vi "database_connection_write_dev_MQTT_database_array_V1.vi"(8 "error in (no error)":errorcluster, 9 "data 2":dbl[](array[numeric]), 10 "Machine Data":T5={"Zload"="", "Yload"="", "Xload"="", "path_position"="", "Fovr"="", "SspeedOvr"="", "Program Name"="", "Program status"="", "Block of code being executed"="", "Line of code"="", "Machine availability"="", "Emergency status"="", "Controller mode"="", "Tool_id"="UNAVAILABLE"}, 11 "current time 2":timestamp) -> (3 "error out":errorcluster)   [LabVIEW 2017]
uses:
  mqtt Folder/src/class/mqtt/mqttTypedef/mqttConnectionStatus.ctl
  mqtt Folder/src/class/mqtt/mqttTypedef/mqttConnectionMeta.ctl
  mqtt Folder/src/class/mqtt/mqttTypedef/mqttQOSlevel.ctl
  data_base_structure_V2.ctl
  mqtt Folder/src/class/mqtt/mqttConfigFunction.ctl
  mqtt Folder/src/class/mqtt/mqttTypedef/mqttBroker.ctl
  mqtt Folder/src/class/mqtt/mqttTypedef/mqttConnectionFlags.ctl
  mqtt Folder/src/class/mqtt/mqttTypedef/mqttWillInformation.ctl
  mqtt Folder/src/class/mqtt/mqttTXqueue/mqttTXdataQueueFunction.ctl
  mqtt Folder/src/class/mqtt/mqttTXqueue/mqttRXsubscriptionEventFunction.ctl
  data_base_structure.ctl
  <vilib>/addons/database/Connection.llb/DB Tools Open Connec (Path).vi
  mqtt Folder/src/class/mqtt/mqtt.lvclass
  <vilib>/addons/database/NI_Database_API.lvlib
panel:
  out "cluster":T1
  out "Xload":string
  out "Machine availability":string
  out "resulting string":string
  out "output array 2":dbl[](array[numeric])
  out "size(s) 2":i32
  out "error out 3":errorcluster
  out "publishSuccess 2":bool=TRUE
  out "publishMessageID 2":u16 format="%02x"
  out "valueSent 2":string="14:19:17.238_"
  in  "connMeta 2":T2
  in  "topic 2":string="a/b"
  out "connStatus 2":T4
  out "sessionPresent 2":bool
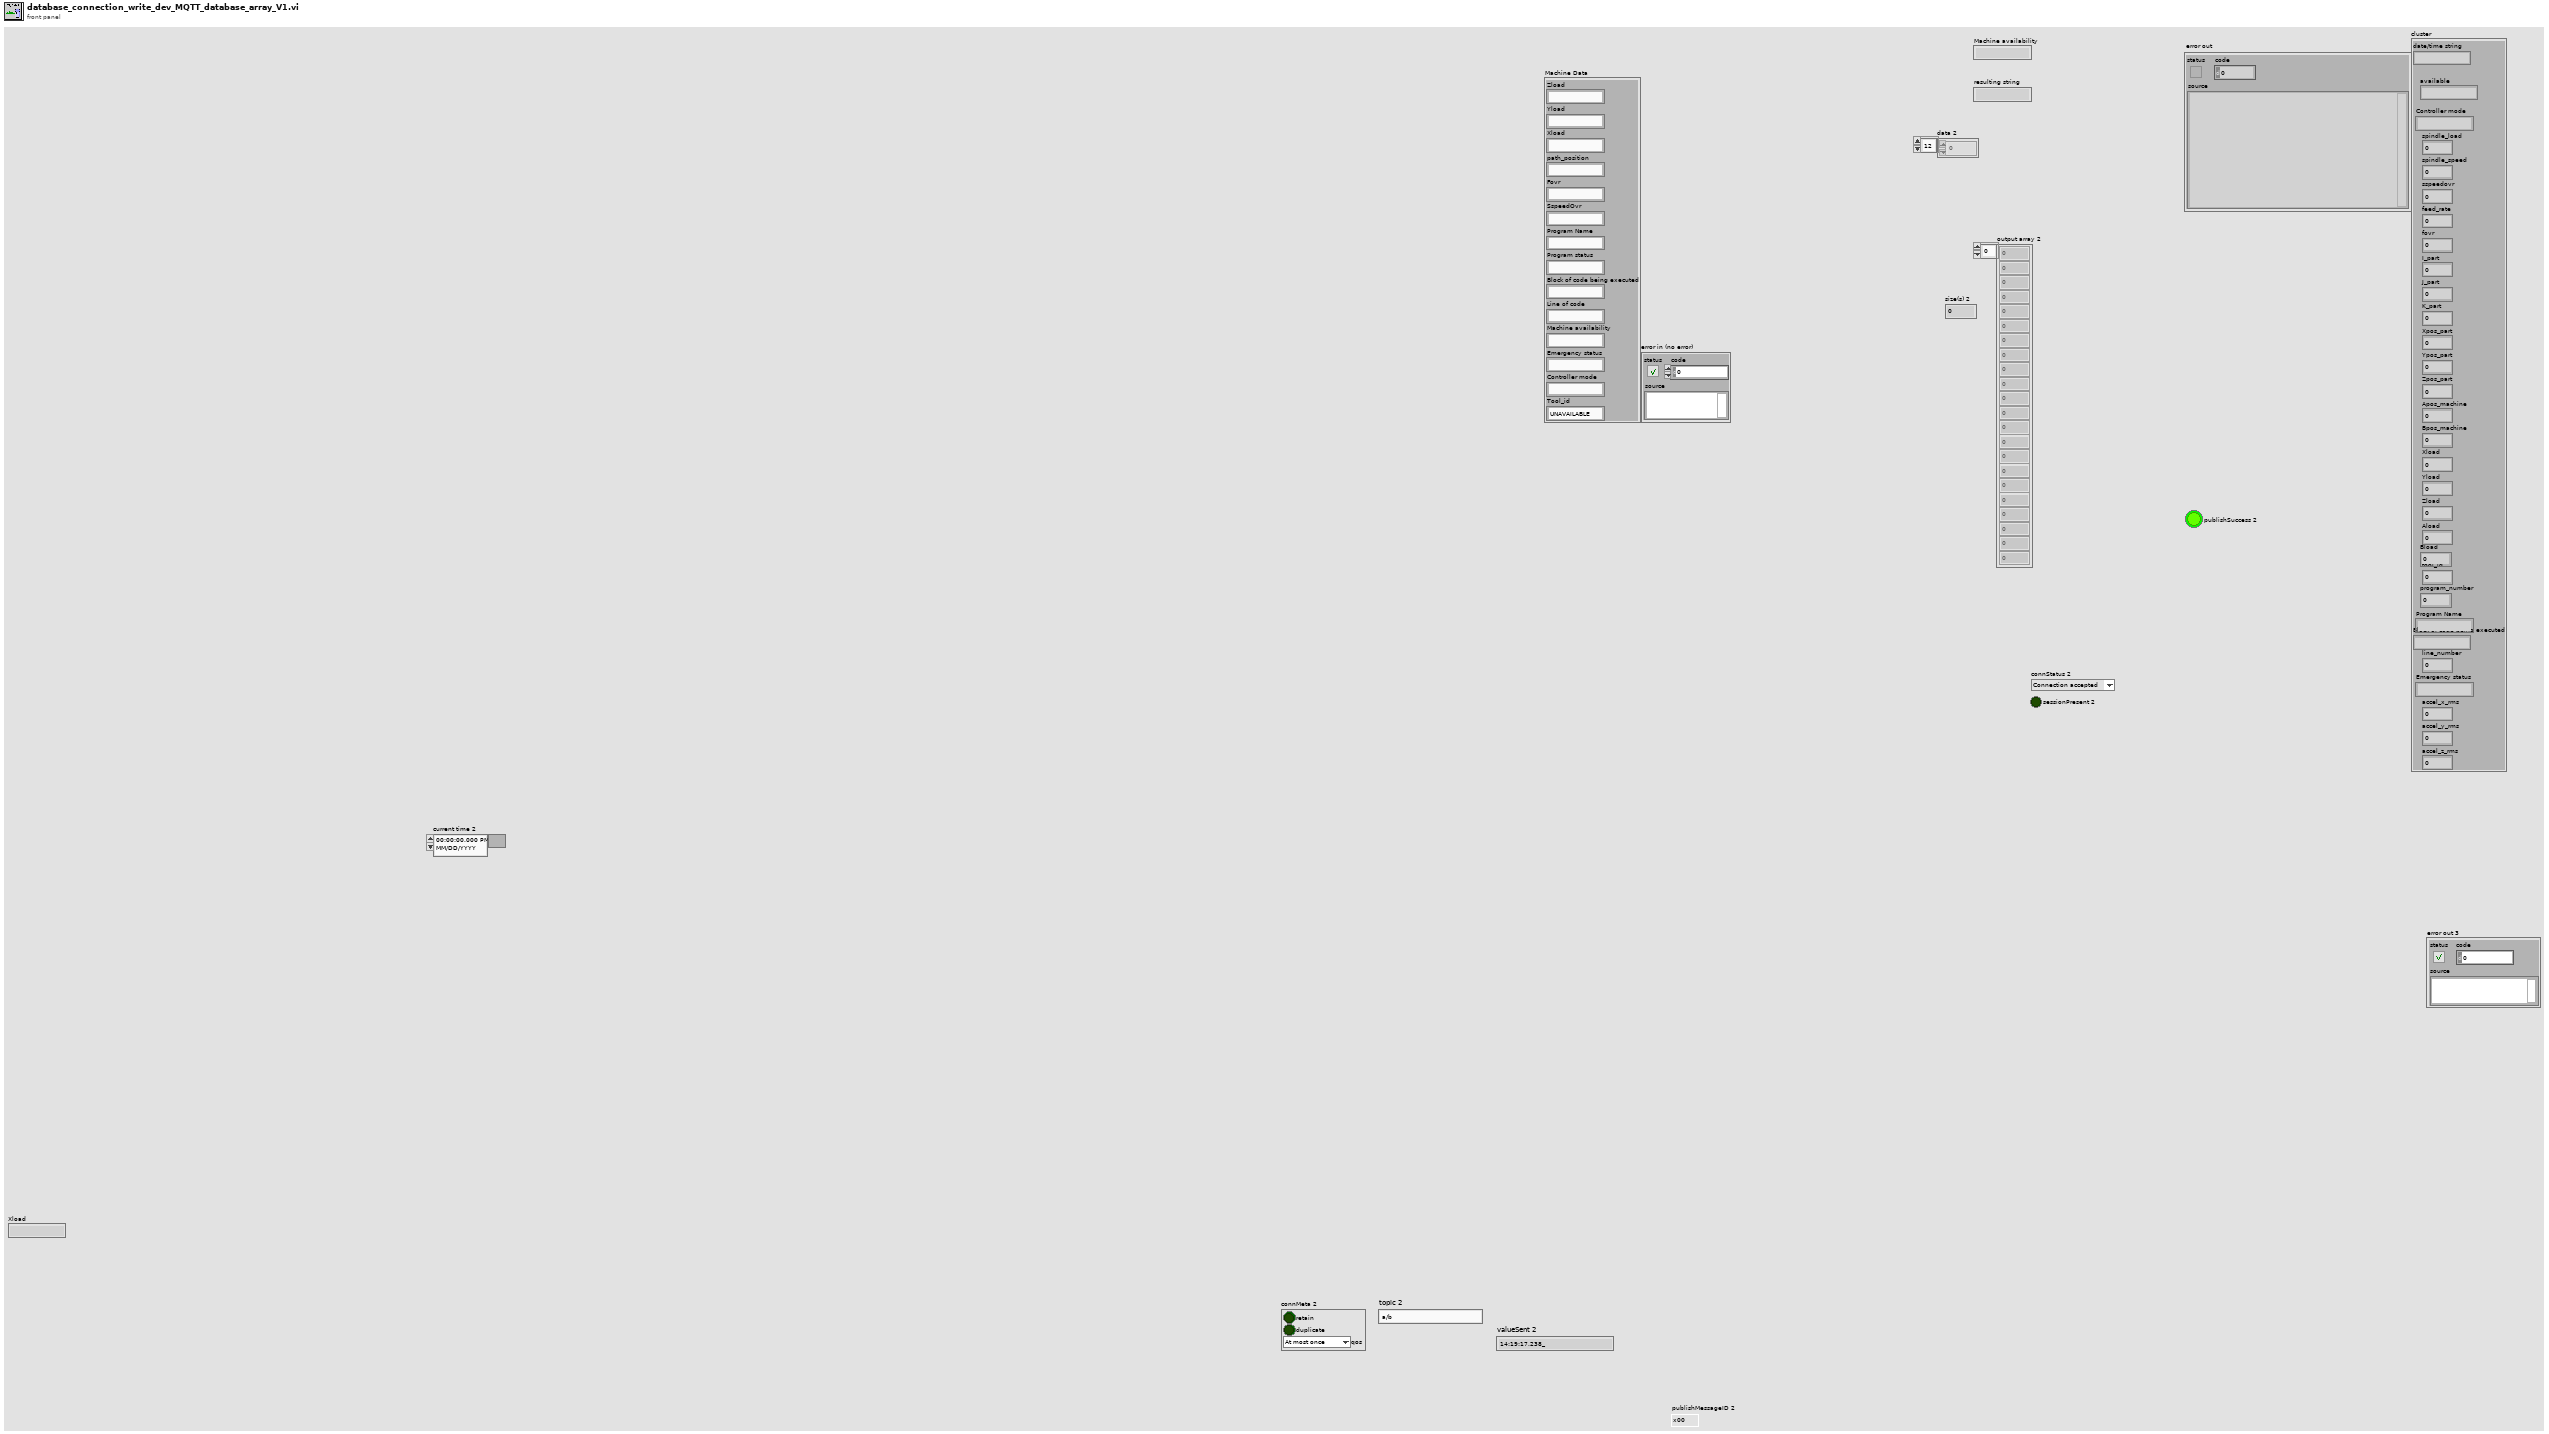
[diagram p1: front panel]
types:
  T1 = typedef "data_base_structure_V2.ctl" = cluster{"date/time string":string, "available":string, "Controller mode":string, "spindle_load":dbl, "spindle_speed":dbl, "sspeedovr":dbl, "feed_rate":dbl, "fovr":dbl, "I_part":dbl, "J_part":dbl, "K_part":dbl, "Xpos_part":dbl, "Ypos_part":dbl, "Zpos_part":dbl, "Apos_machine":dbl, "Bpos_machine":dbl, "Xload":dbl, "Yload":dbl, "Zload":dbl, "Aload":dbl, "Bload":dbl, "tool_id":dbl, "program_number":dbl, "Program Name":string, "Block of code being executed":string, "line_number":dbl, "Emergency status":string, "accel_x_rms":dbl, "accel_y_rms":dbl, "accel_z_rms":dbl}
  T2 = typedef "mqttConnectionMeta.ctl" = cluster{"retain":bool, "duplicate":bool, "qos":T3}
  T3 = typedef "mqttQOSlevel.ctl" = enum8{"At most once", "At least once", "Exactly once", "Reserved"}
  T4 = typedef "mqttConnectionStatus.ctl" = enum16{"Connection accepted", "Connection refused: unacceptable protocol version", "Connection refused: identifier rejected", "Connection refused: Server unavailable", "Connection refused: bad user name or password", "Connection refused: not authorized"}
  T5 = cluster{"Zload":string, "Yload":string, "Xload":string, "path_position":string, "Fovr":string, "SspeedOvr":string, "Program Name":string, "Program status":string, "Block of code being executed":string, "Line of code":string, "Machine availability":string, "Emergency status":string, "Controller mode":string, "Tool_id":string}
  T6 = typedef "data_base_structure.ctl" = cluster{"available ":dbl, "controller_mode":string, "spindle_load":dbl, "spindle_speed ":dbl, "sspeedovr":dbl, "J_part":dbl, "K_part":dbl, "Xpos_part":dbl, "Ypos_part":dbl, "Zpos_part":dbl, "Apos_machine":dbl, "Bpos_machine":dbl, "Xload":dbl, "Yload":dbl, "Zload":dbl, "Aload":dbl, "Bload":dbl, "tool_id":dbl, "program_name":string, "block_code":string, "line_number":dbl, "estop":string, "accel_x_rms":dbl, "accel_y_rms":dbl, "accel_z_rms":dbl, "program_number":dbl, "timestamp":string, "feed_rate ":dbl, "fovr":dbl, "I_part ":dbl}
  T7 = typedef "mqttRXsubscriptionEventFunction.ctl" = enum16{"init", "deinit", "getEventRef", "event"}
  T8 = typedef "mqttTXdataQueueFunction.ctl" = enum16{"init", "deinit", "getQueue", "enqueue"}
  T9 = typedef "mqttWillInformation.ctl" = cluster{"User Name":string, "Password":string}
  T10 = typedef "mqttConnectionFlags.ctl" = cluster{"reserved":bool, "clean session":bool, "will flag":bool, "willQOS":enum8{"At most once", "At least once", "Exactly once", "Reserved"}, "will retain":bool, "password":bool, "user name":bool}
  T11 = typedef "mqttBroker.ctl" = cluster{"address":string, "port":u16, "connTimeout":i32, "writeTimeout":i32, "readTimeout":i32, "subTimeout":i32}
  T12 = typedef "mqtt.lvclass/mqttConfigFunction.ctl" = enum16{"init", "deinit", "set", "get"}
  T13 = enum8{"Enabled", "Disabled", "Disabled and Grayed Out"}
  T14 = cluster{"data 2[0]":dbl, "data 2[1]":dbl, "data 2[2]":dbl, "data 2[3]":dbl, "data 2[4]":dbl, "data 2[5]":dbl, "data 2[6]":dbl, "data 2[7]":dbl, "data 2[8]":dbl, "data 2[9]":dbl, "data 2[10]":dbl, "data 2[11]":dbl, "data 2[12]":dbl, "data 2[13]":dbl, "data 2[14]":dbl, "data 2[15]":dbl, "data 2[16]":dbl, "data 2[17]":dbl, "data 2[18]":dbl, "data 2[19]":dbl, "data 2[20]":dbl, "data 2[21]":dbl}
  T15 = typedef "NI_Database_API.lvlib/Conn ObjectReference.ctl" = refnum<k1>
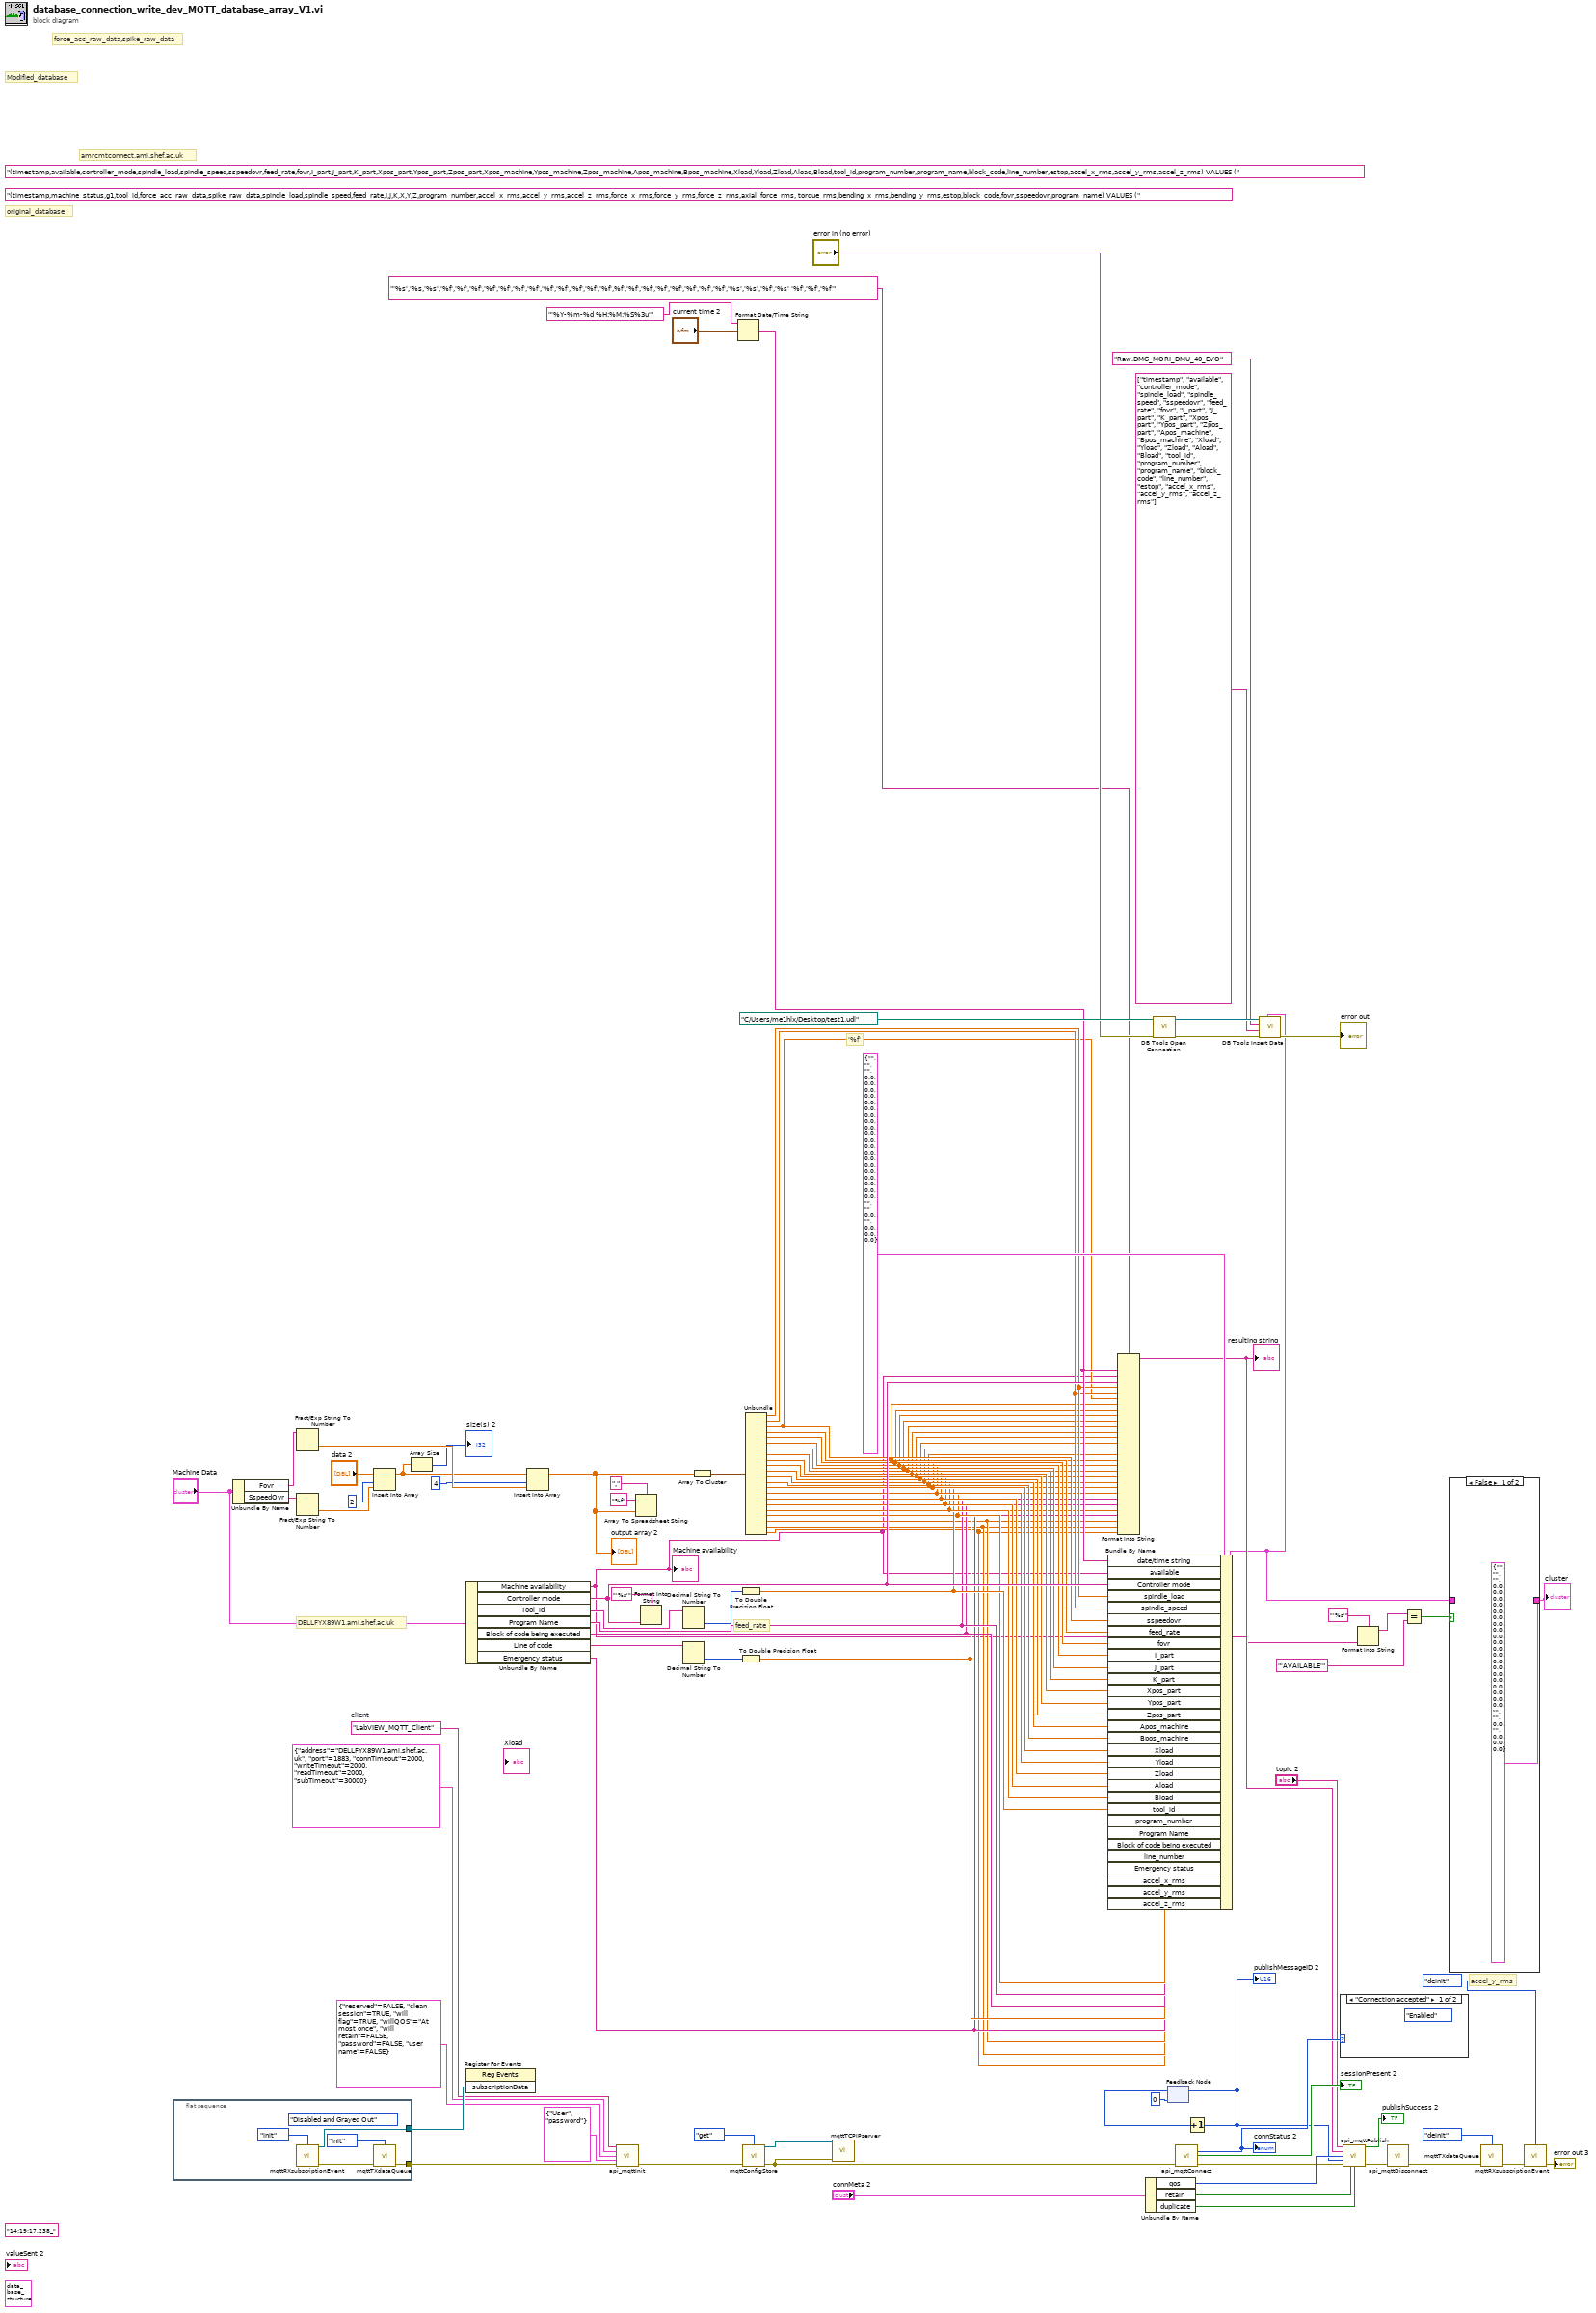
[diagram p0: block diagram]
diagram:
  (unwired) "14:19:17.238_" ("valueSent 2")
  (unwired) T6 {"available "=0.0, "controller_mode"="", "spindle_load"=0.0, "spindle_speed "=0.0, "sspeedovr"=0.0, "J_part"=0.0, "K_part"=0.0, "Xpos_part"=0.0, "Ypos_part"=0.0, "Zpos_part"=0.0, "Apos_machine"=0.0, "Bpos_machine"=0.0, "Xload"=0.0, "Yload"=0.0, "Zload"=0.0, "Aload"=0.0, "Bload"=0.0, "tool_id"=0.0, "program_name"="", "block_code"="", "line_number"=0.0, "estop"="", "accel_x_rms"=0.0, "accel_y_rms"=0.0, "accel_z_rms"=0.0, "program_number"=0.0, "timestamp"="", "feed_rate "=0.0, "fovr"=0.0, "I_part "=0.0} ("Cluster")
  (unwired) "(timestamp,available,controller_mode,spindle_load,spindle_speed,sspeedovr,feed_rate,fovr,I_part,J_part,K_part,Xpos_part,Ypos_part,Zpos_part,Xpos_machine,Ypos_machine,Zpos_machine,Apos_machine,Bpos_machine,Xload,Yload,Zload,Aload,Bload,tool_id,program_number,program_name,block_code,line_number,estop,accel_x_rms,accel_y_rms,accel_z_rms) VALUES (" ("string")
  w88 = "LabVIEW_MQTT_Client"  # client
  (unwired) "(timestamp,machine_status,g1,tool_id,force_acc_raw_data,spike_raw_data,spindle_load,spindle_speed,feed_rate,I,J,K,X,Y,Z,program_number,accel_x_rms,accel_y_rms,accel_z_rms,force_x_rms,force_y_rms,force_z_rms,axial_force_rms, torque_rms,bending_x_rms,bending_y_rms,estop,block_code,fovr,sspeedovr,program_name) VALUES (" ("string")
  # "'%f'"
  # "accel_y_rms"
  # "feed_rate"
  # "original_database"
  # "force_acc_raw_data,spike_raw_data"
  # "Modified_database"
  # "amrcmtconnect.ami.shef.ac.uk"
  # "DELLFYX89W1.ami.shef.ac.uk"
  n1 = flat-sequence {
    tunnel: [w99] -> w93
    tunnel: [w96] -> w89
    frame #0 {
      (unwired) T13."Disabled and Grayed Out" ("Disabled")
      n2 = call "mqttRXsubscriptionEvent.vi"("function"=mqttRXsubscriptionEventFunction."init") -> ("subscriptionData"=w96:refnum<user-event>, "error out"=w98:errorcluster)  [unwired: 13 in]
      n3 = call "mqttTXdataQueue.vi"("function"=mqttTXdataQueueFunction."init", "error in (no error)"=w98) -> ("error out"=w99:errorcluster)  [unwired: 12 in, 1 out]
    }
  }
  n4 = Unbundle By Name("Machine Data") -> ("Fovr"=w59:string, "SspeedOvr"=w64:string)
  n5 = Fract/Exp String To Number(string=w59) -> (number=w61:dbl)  [unwired: 3 in, 1 out]
  n6 = Fract/Exp String To Number(string=w64) -> (number=w63:dbl)  [unwired: 3 in, 1 out]
  n7 = Insert Into Array(array="data 2", index=2, new element=w63) -> (w52:dbl[])
  n8 = Array Size(array=w52) -> (size(s)=→"size(s) 2":i32)
  n9 = Unbundle By Name("Machine Data") -> ("Machine availability"=w5:string, "Controller mode"=w37:string, "Tool_id"=w49:string, "Program Name"=w16:string, "Block of code being executed"=w15:string, "Line of code"=w48:string, "Emergency status"=w13:string)
  "Machine availability" <- w5
  n10 = register-events(w89) -> ()  [unwired: 2 in, 2 out]
  n11 = Insert Into Array(array=w52, index=4, new element=w61) -> (w42:dbl[])
  "output array 2" <- w42
  n12 = call "api_mqttInit.vi"("client"=w88, "broker"=T11 {"address"="DELLFYX89W1.ami.shef.ac.uk", "port"=1883, "connTimeout"=2000, "writeTimeout"=2000, "readTimeout"=2000, "subTimeout"=30000}, "connFlags"=T10 {"reserved"=FALSE, "clean session"=TRUE, "will flag"=TRUE, "willQOS"=enum."At most once", "will retain"=FALSE, "password"=FALSE, "user name"=FALSE}, "User Info"=T9 {"User Name"="User", "Password"="password"}, "error in (no error)"=w93) -> ("error out"=w91:errorcluster)  [unwired: 10 in]
  n13 = Array To Spreadsheet String(delimiter (Tab)=",", array=w42, 3:"%f" ("format string")) -> ()  [unwired: 1 out]
  n14 = Format Into String(format string="'%s'", w37) -> ()  [unwired: 2 in, 2 out]
  n15 = Decimal String To Number(string=w49) -> (number=w50:i32)  [unwired: 2 in, 1 out]
  n16 = Decimal String To Number(string=w48) -> (number=w47:i32)  [unwired: 2 in, 1 out]
  n17 = Array To Cluster(array=w42) -> (cluster=w41:T14)
  n18 = Format Date/Time String(time format string (%c)="'%Y-%m-%d %H:%M:%S%3u'", seconds (now)="current time 2") -> (date/time string=w38:string)  [unwired: 1 in]
  n19 = To Double Precision Float(number=w50) -> (double precision float=w18:dbl)
  n20 = To Double Precision Float(number=w47) -> (double precision float=w14:dbl)
  n21 = call "mqttConfigStore.vi"("function"=mqttConfigFunction."get", "error in (no error)"=w91) -> ("mqtt.lvclass out"=w90:refnum<class "mqtt.lvclass">, "error out"=w82:errorcluster)  [unwired: 12 in]
  n22 = Unbundle(w41) -> ("data 2[0]"=w36:dbl, "data 2[1]"=w35:dbl, "data 2[2]"=w34:dbl, "data 2[3]"=w33:dbl, "data 2[4]"=w32:dbl, "data 2[5]"=w31:dbl, "data 2[6]"=w30:dbl, "data 2[7]"=w29:dbl, "data 2[8]"=w28:dbl, "data 2[9]"=w27:dbl, "data 2[10]"=w26:dbl, "data 2[11]"=w25:dbl, "data 2[12]"=w24:dbl, "data 2[13]"=w23:dbl, "data 2[14]"=w22:dbl, "data 2[15]"=w21:dbl, "data 2[16]"=w20:dbl, "data 2[17]"=w19:dbl, "data 2[18]"=w17:dbl, "data 2[19]"=w11:dbl, "data 2[20]"=w10:dbl, "data 2[21]"=w9:dbl)
  n23 = call "mqttTCPIPserver.vi"("mqtt.lvclass"=w90, "error in (no error)"=w82) -> ()  [unwired: 12 in, 2 out]
  n24 = Bundle By Name(cluster=T1 {"date/time string"="", "available"="", "Controller mode"="", "spindle_load"=0.0, "spindle_speed"=0.0, "sspeedovr"=0.0, "feed_rate"=0.0, "fovr"=0.0, "I_part"=0.0, "J_part"=0.0, "K_part"=0.0, "Xpos_part"=0.0, "Ypos_part"=0.0, "Zpos_part"=0.0, "Apos_machine"=0.0, "Bpos_machine"=0.0, "Xload"=0.0, "Yload"=0.0, "Zload"=0.0, "Aload"=0.0, "Bload"=0.0, "tool_id"=0.0, "program_number"=0.0, "Program Name"="", "Block of code being executed"="", "line_number"=0.0, "Emergency status"="", "accel_x_rms"=0.0, "accel_y_rms"=0.0, "accel_z_rms"=0.0}, "date/time string"=w38, "available"=w5, "Controller mode"=w37, "spindle_load"=w36, "spindle_speed"=w35, "sspeedovr"=w34, "feed_rate"=w33, "fovr"=w32, "I_part"=w31, "J_part"=w30, "K_part"=w29, "Xpos_part"=w28, "Ypos_part"=w27, "Zpos_part"=w26, "Apos_machine"=w25, "Bpos_machine"=w24, "Xload"=w23, "Yload"=w22, "Zload"=w21, "Aload"=w20, "Bload"=w19, "tool_id"=w18, "program_number"=w17, "Program Name"=w16, "Block of code being executed"=w15, "line_number"=w14, "Emergency status"=w13, "accel_x_rms"=w11, "accel_y_rms"=w10, "accel_z_rms"=w9) -> (w2:T1)
  n25 = Format Into String(format string="'%s','%s,'%s','%f','%f','%f','%f','%f','%f','%f','%f','%f','%f','%f','%f',%f','%f','%f','%f','%f','%f','%f','%f','%s','%s','%f','%s' '%f','%f','%f'", w38, w5, w37, w36, w35, w34, w33, w32, w31, w30, w29, w28, w27, w26, w25, w24, w23, w22, w21, w20, w19, w18, w17, w16, w15, w14, w13, w11, w10, w9) -> (resulting string=w8:string)  [unwired: 2 in, 1 out]
  "resulting string" <- w8
  n26 = Unbundle By Name("connMeta 2") -> ("qos"=w79:T3, "retain"=w78:bool, "duplicate"=w77:bool)
  n27 = call-poly <vilib>:"DB Tools Open Connection.vi"("error in (no error)"="error in (no error)", "connection information"=path "C:/Users/me1hlx/Desktop/test1.udl") -> ("error out"=w51:errorcluster, "connection reference"=w56:T15)  [unwired: 6 in]
  n28 = feedback #1(u16 0) -> (w74:u16)
  n29 = call "api_mqttConnect.vi"("error in (no error)"=w82) -> ("connStatus"=w84:T4, "sessionPresent"=→"sessionPresent 2":bool, "error out"=w76:errorcluster)  [unwired: 11 in, 1 out]
  "connStatus 2" <- w84
  n30 = Increment(x=w74) -> (x+1=w73:u16)
  "publishMessageID 2" <- w73
  n31 = feedback-in #1(w73) -> ()
  n32 = call <vilib>:"DB Tools Insert Data.vi"("data"=w2, "error in (no error)"=w51, "columns"=string[] ["timestamp", "available", "controller_mode", "spindle_load", "spindle_speed", "sspeedovr", "feed_rate", "fovr", "I_part", "J_part", "K_part", "Xpos_part", "Ypos_part", "Zpos_part", "Apos_machine", "Bpos_machine", "Xload", "Yload", "Zload", "Aload", "Bload", "tool_id", "program_number", "program_name", "block_code", "line_number", "estop", "accel_x_rms", "accel_y_rms", "accel_z_rms"], "table"="Raw.DMG_MORI_DMU_40_EVO" ("string"), "connection reference"=w56) -> ("error out"=→"error out":errorcluster)  [unwired: 5 in, 1 out]
  n33 = case shown="\"Connection accepted\"" w84 {
    frame "Connection accepted" {
      (unwired) T13."Enabled" ("Disabled")
    }
    frame Default {
    }
  }
  n34 = call "api_mqttPublish.vi"("topic"="topic 2", "value"=w8, "QoS (At most once)"=w79, "messageID"=w73, "error in (no error)"=w76, "retain(F)"=w78, "duplicate(F)"=w77) -> ("success"=→"publishSuccess 2":bool, "error out"=w66:errorcluster)  [unwired: 7 in]
  n35 = Format Into String(format string="'%s'", w5) -> (resulting string=w6:string)  [unwired: 2 in, 1 out]
  n36 = call "api_mqttDisconnect.vi"("error in (no error)"=w66) -> ("error out"=w70:errorcluster)  [unwired: 13 in, 1 out]
  n37 = Equal?(x=w6, y="'AVAILABLE'") -> (x = y?=w3:bool)
  n38 = case shown="False" w3 {
    tunnel: w2 -> [_ w102]
    tunnel: [T1 {"date/time string"="", "available"="", "Controller mode"="", "spindle_load"=0.0, "spindle_speed"=0.0, "sspeedovr"=0.0, "feed_rate"=0.0, "fovr"=0.0, "I_part"=0.0, "J_part"=0.0, "K_part"=0.0, "Xpos_part"=0.0, "Ypos_part"=0.0, "Zpos_part"=0.0, "Apos_machine"=0.0, "Bpos_machine"=0.0, "Xload"=0.0, "Yload"=0.0, "Zload"=0.0, "Aload"=0.0, "Bload"=0.0, "tool_id"=0.0, "program_number"=0.0, "Program Name"="", "Block of code being executed"="", "line_number"=0.0, "Emergency status"="", "accel_x_rms"=0.0, "accel_y_rms"=0.0, "accel_z_rms"=0.0} ("cluster") w102] -> w1
    frame False {
    }
    frame True {
    }
  }
  "cluster" <- w1
  n39 = call "mqttTXdataQueue.vi"("function"=mqttTXdataQueueFunction."deinit", "error in (no error)"=w70) -> ("error out"=w68:errorcluster)  [unwired: 12 in, 1 out]
  n40 = call "mqttRXsubscriptionEvent.vi"("function"=mqttRXsubscriptionEventFunction."deinit", "error in (no error)"=w68) -> ("error out"=→"error out 3":errorcluster)  [unwired: 12 in, 1 out]
